vi "UI_Method.vi"(0 "Object In":refnum<class "Arithmetic_Operations.lvclass">, 5 "Num 1":dbl, 7 "Num 2":dbl, 11 "Error In":errorcluster) -> (4 "Object Out":refnum<class "Arithmetic_Operations.lvclass">, 6 "Output":dbl, 15 "Error Out":errorcluster)   [LabVIEW 2020]
uses:
  Arithmetic_Operations.lvclass
  Typedef's/UserEvent_Operations.ctl
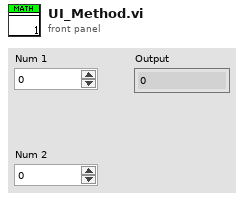
[diagram p1: front panel]
types:
  T1 = typedef "UserEvent_Operations.ctl" = enum16{"Create", "Generate", "Get Ref", "Destroy"}
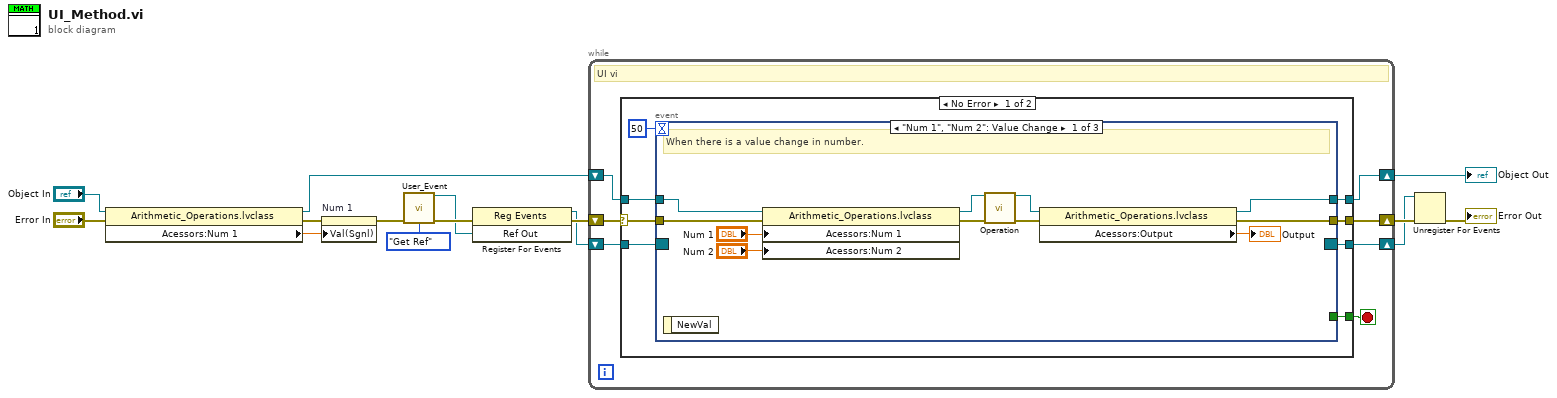
[diagram p0: block diagram]
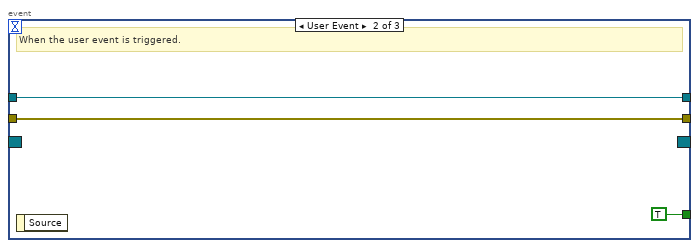
[diagram p2: hidden frame]
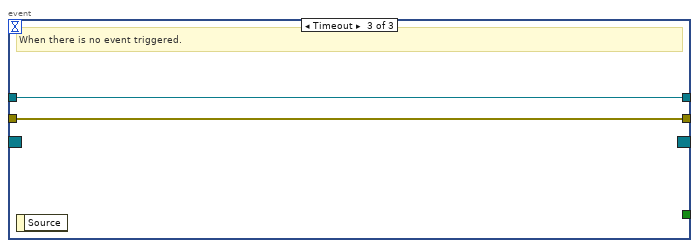
[diagram p3: hidden frame]
diagram:
  n1 = property class="Arithmetic_Operations.lvclass"(reference="Object In", error in="Error In") -> (reference out=w3:refnum<class "Arithmetic_Operations.lvclass">, error out=w5:errorcluster, "Acessors:Num 1"=w1:dbl)
  n2 = property on="Num 1" class="DigNum (strict)"(error in=w5, "Val(Sgnl)"=w1) -> (error out=w2:errorcluster)  [unwired: 1 in, 1 out]
  n3 = call "User_Event.vi"("Error In"=w2, "Enum"=UserEvent_Operations."Get Ref") -> ("Ref Out"=w9:refnum<user-event>, "Error Out"=w12:errorcluster)  [unwired: 12 in]
  n4 = register-events(error in=w12, w9) -> (reference out=w8:refnum<event-registration>, error out=w10:errorcluster)  [unwired: 1 in]
  n5 = while {
    shift-right: [w21] -> w14
    shift-left: w10 -> [w22]
    shift-right: [w19] -> w13
    shift-left: w3 -> [w20]
    shift-right: [w17] -> w6
    shift-left: w8 -> [w18]
    stop <- w16 stop-if-true
    # "UI vi"
    n6 = case shown="No Error" w22 {
      selector: w22 -> [w29 w49]
      tunnel: [w28 w49] -> w21
      tunnel: [w27 w48] -> w19
      tunnel: w20 -> [w30 w48]
      tunnel: w18 -> [w25 w47]
      tunnel: [w24 w47] -> w17
      tunnel: [w23 _] -> w16
      frame No Error {
        n7 = event shown="[0] \"Num 1\", \"Num 2\": Value Change" {
          selector: w25 -> [_ _ _]
          dyn-events: [_ _ _] -> w24
          timeout: 50 -> [_ _ _]
          tunnel: w30 -> [w41 w43 w46]
          tunnel: w29 -> [w40 w44 w45]
          tunnel: [w36 w44 w45] -> w28
          tunnel: [w34 w43 w46] -> w27
          tunnel: [_ TRUE _] -> w23
          event "Num 1", "Num 2": Value Change {
            # "When there is a value change in number."
            n8 = event-data() -> ()  [unwired: 1 in, 1 out]
            n9 = property class="Arithmetic_Operations.lvclass"(reference=w41, error in=w40, "Acessors:Num 1"="Num 1", "Acessors:Num 2"="Num 2") -> (reference out=w39:refnum<class "Arithmetic_Operations.lvclass">, error out=w38:errorcluster)
            n10 = call-dynamic "Operation.vi"("Arithmetic_Operations in"=w39, "Error In"=w38) -> ("Arithmetic_Operations out"=w35:refnum<class "Arithmetic_Operations.lvclass">, "Error Out"=w37:errorcluster)  [unwired: 12 in]
            n11 = property class="Arithmetic_Operations.lvclass"(reference=w35, error in=w37) -> (reference out=w34:refnum<class "Arithmetic_Operations.lvclass">, error out=w36:errorcluster, "Acessors:Output"=→"Output":dbl)
          }
          event User Event {
            # "When the user event is triggered."
            n12 = event-data() -> ()  [unwired: 1 in, 1 out]
          }
          event Timeout {
            # "When there is no event triggered."
            n13 = event-data() -> ()  [unwired: 1 in, 1 out]
          }
        }
      }
      frame Error {
      }
    }
  }
  "Object Out" <- w13
  n14 = Unregister For Events(event registration refnum=w6, error in=w14) -> (error out=→"Error Out":errorcluster)
